vi "GuideRate.vi"(7 "Guide Rate":dbl=0.01 min=0.01 max=3.0 step=0.01 format="%.2f") -> (8 "Guide Rate out":dbl format="%.1f")   [LabVIEW 2011]
panel:
  in  "cancel":bool
  in  "acceot":bool
  # "\"/s"
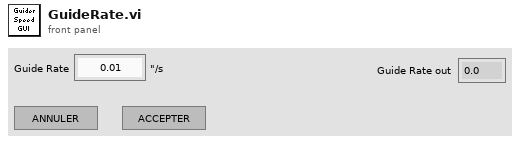
[diagram p1: front panel]
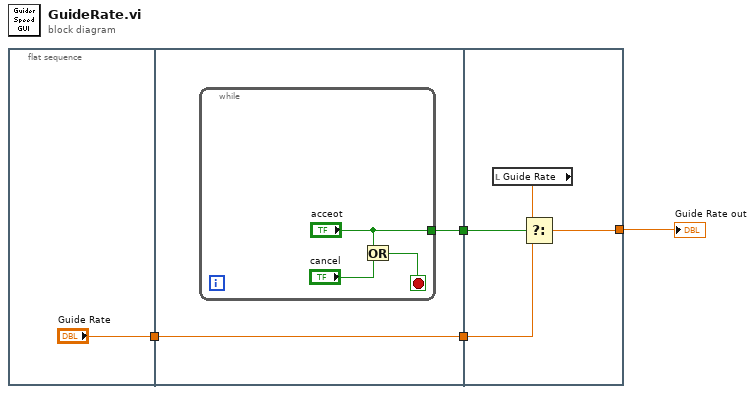
[diagram p0: block diagram]
diagram:
  n1 = flat-sequence {
    tunnel: ["Guide Rate"] -> w4
    tunnel: w4 -> [w6]
    tunnel: [w7] -> w3
    tunnel: [w6] -> w2
    tunnel: w3 -> [w14]
    tunnel: w2 -> [w13]
    tunnel: [w11] -> w1
    frame #0 {
    }
    frame #1 {
      n2 = while {
        tunnel: ["acceot"] -> w7
        stop <- w9 stop-if-true
        n3 = Or(x="acceot", y="cancel") -> (x .or. y?=w9:bool)
      }
    }
    frame #2 {
      n4 = local read "Guide Rate"() -> (w12:dbl)
      n5 = Select(t=w12, s=w14, f=w13) -> (s? t:f=w11:dbl)
    }
  }
  "Guide Rate out" <- w1
